vi "getDevice.vi"(1 "starting_string":string, 2 "data":string) -> (0 "deviceString":string)   [LabVIEW 2010]
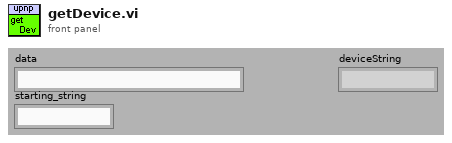
[diagram p1: front panel]
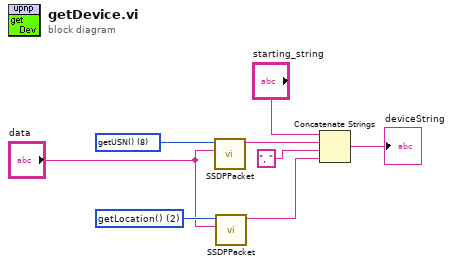
[diagram p0: block diagram]
diagram:
  w7 = u16 2 items=["getHost()", "getCacheControl()", "getLocation()", "getMAN()", "getST()", "getNT()", "getNTS()", "getServer()", "getUSN()", "getMX()"] ("getMethods")
  w8 = u16 8 items=["getHost()", "getCacheControl()", "getLocation()", "getMAN()", "getST()", "getNT()", "getNTS()", "getServer()", "getUSN()", "getMX()"] ("getMethods")
  n1 = call "SSDPPacket.vi"("data"="data", "getMethods"=w8) -> ("value"=w5:string)  [unwired: 9 out]
  n2 = call "SSDPPacket.vi"("data"="data", "getMethods"=w7) -> ("value"=w1:string)  [unwired: 9 out]
  n3 = Concatenate Strings("starting_string", w5, ", ", w1) -> (→"deviceString":string)
